vi "Keithley617_Configure_IV.vi"(7 "GPIB Address String":string="27", 8 "Error In":errorcluster) -> (0 "Error Out":errorcluster)   [LabVIEW 2015, in "Keithley617.lvlib"]
uses:
  Keithley617.lvlib
  Keithley617_GPIB_Commands.ctl
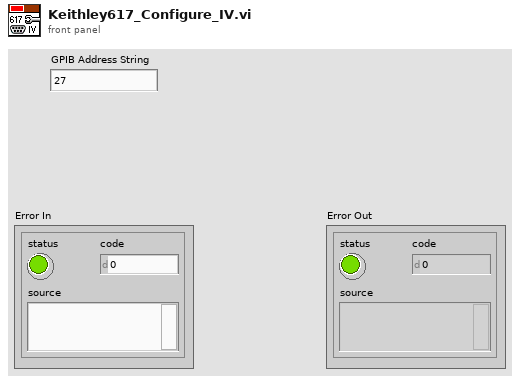
[diagram p1: front panel]
types:
  T1 = typedef "Keithley617_GPIB_Commands.ctl" = string
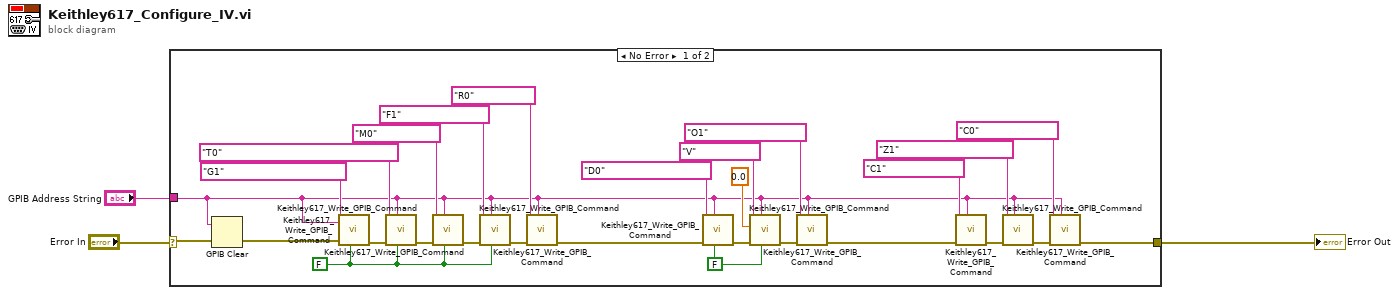
[diagram p0: block diagram]
diagram:
  n1 = case shown="No Error" "Error In" {
    selector: "Error In" -> [w8 w32]
    tunnel: [w9 w32] -> w2
    tunnel: "GPIB Address String" -> [w6 _]
    frame No Error {
      w4 = FALSE ("Execute Command?")
      w5 = FALSE ("Execute Command?")
      n2 = GPIB Clear(2:w8, 3:w6) -> (0:w7:errorcluster)  [unwired: 1 out]
      n3 = call "Keithley617_Write_GPIB_Command.vi"("Execute Command?"=w4, "GPIB Address String"=w6, "Error In"=w7, "Command"=T1 "G1") -> ("Error Out"=w29:errorcluster)  [unwired: 7 in]
      n4 = call "Keithley617_Write_GPIB_Command.vi"("Execute Command?"=w4, "GPIB Address String"=w6, "Error In"=w29, "Command"=T1 "T0") -> ("Error Out"=w31:errorcluster)  [unwired: 7 in]
      n5 = call "Keithley617_Write_GPIB_Command.vi"("Execute Command?"=w4, "GPIB Address String"=w6, "Error In"=w31, "Command"=T1 "M0") -> ("Error Out"=w28:errorcluster)  [unwired: 7 in]
      n6 = call "Keithley617_Write_GPIB_Command.vi"("Execute Command?"=w4, "GPIB Address String"=w6, "Error In"=w28, "Command"=T1 "F1") -> ("Error Out"=w30:errorcluster)  [unwired: 7 in]
      n7 = call "Keithley617_Write_GPIB_Command.vi"("GPIB Address String"=w6, "Error In"=w30, "Command"=T1 "R0") -> ("Error Out"=w25:errorcluster)  [unwired: 8 in]
      n8 = call "Keithley617_Write_GPIB_Command.vi"("Execute Command?"=w5, "GPIB Address String"=w6, "Error In"=w25, "Command"=T1 "D0") -> ("Error Out"=w26:errorcluster)  [unwired: 7 in]
      n9 = call "Keithley617_Write_GPIB_Command.vi"("Execute Command?"=w5, "GPIB Address String"=w6, "Error In"=w26, "Value"=0.0, "Command"=T1 "V") -> ("Error Out"=w27:errorcluster)  [unwired: 6 in]
      n10 = call "Keithley617_Write_GPIB_Command.vi"("GPIB Address String"=w6, "Error In"=w27, "Command"=T1 "O1") -> ("Error Out"=w24:errorcluster)  [unwired: 8 in]
      n11 = call "Keithley617_Write_GPIB_Command.vi"("GPIB Address String"=w6, "Error In"=w24, "Command"=T1 "C1") -> ("Error Out"=w22:errorcluster)  [unwired: 8 in]
      n12 = call "Keithley617_Write_GPIB_Command.vi"("GPIB Address String"=w6, "Error In"=w22, "Command"=T1 "Z1") -> ("Error Out"=w23:errorcluster)  [unwired: 8 in]
      n13 = call "Keithley617_Write_GPIB_Command.vi"("GPIB Address String"=w6, "Error In"=w23, "Command"=T1 "C0") -> ("Error Out"=w9:errorcluster)  [unwired: 8 in]
    }
    frame Error {
    }
  }
  "Error Out" <- w2
